vi "LoadFDC.vi"(11 "file path (use dialog)":path=path "C:/Users/appli/Documents/Manip Gaz/Moteurs manip Gaz/PilMOT/RefsMoteurs/FDC.dat") -> (0 "error out":errorcluster, 1 "FDC+":i32[](array[numeric]), 2 "FDC-":i32[](array[numeric]))   [LabVIEW 2013]
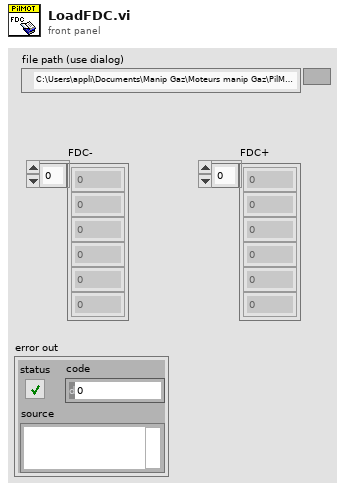
[diagram p1: front panel]
types:
  T1 = enum16{"open", "replace", "create", "open or create", "replace or create", "replace or create with confirmation"}
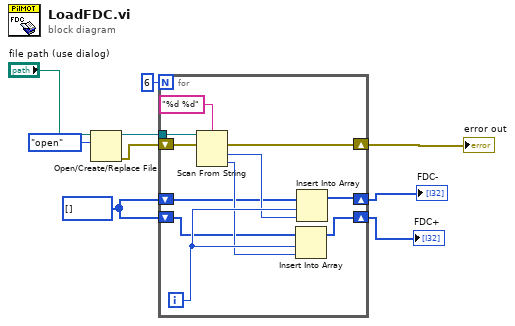
[diagram p0: block diagram]
diagram:
  w4 = i32[] [] ("array")
  n1 = Open/Create/Replace File(file path (use dialog)="file path (use dialog)", operation (0:open)=T1."open") -> (refnum out=w7:refnum<file>, error out=w6:errorcluster)  [unwired: 4 in, 1 out]
  n2 = for {
    N: 6 -> [_]
    tunnel: w7 -> [w20]
    shift-right: [w12] -> w3
    shift-left: w4 -> [w14]
    shift-right: [w11] -> w2
    shift-left: w4 -> [w13]
    shift-right: [w10] -> w1
    shift-left: w6 -> [w19]
    i -> [w17]
    n3 = Scan From String("%d %d" ("format string"), w20, w19) -> (w10:errorcluster, output 1=w16:i32, output 2=w15:i32)  [unwired: 2 in, 1 out]
    n4 = Insert Into Array(array=w13, index=w17, new element=w15) -> (w11:i32[])
    n5 = Insert Into Array(array=w14, index=w17, new element=w16) -> (w12:i32[])
  }
  "FDC-" <- w3
  "FDC+" <- w2
  "error out" <- w1
